vi "To String.vi"(8 "error in (no error)":errorcluster, 11 "BuildWorker in":refnum<class "BuildWorker.lvclass">) -> (0 "error out":errorcluster, 2 "String":string, 3 "BuildWorker out":refnum<class "BuildWorker.lvclass">)   [LabVIEW 2017, in "BuildWorker Interface.lvlib" / "BuildWorker.lvclass"]
uses:
  BuildWorker.lvclass
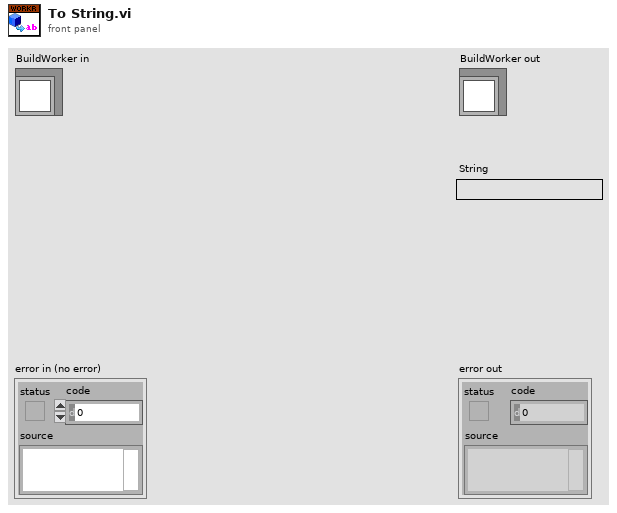
[diagram p1: front panel]
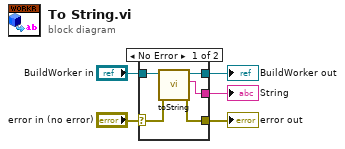
[diagram p0: block diagram]
diagram:
  n1 = case shown="No Error" "error in (no error)" {
    selector: "error in (no error)" -> [w8 w12]
    tunnel: [w7 w12] -> w4
    tunnel: [w9 w11] -> w2
    tunnel: "BuildWorker in" -> [w10 w11]
    tunnel: [w6 _] -> w1
    frame No Error {
      n2 = call-dynamic "toString.vi"("error in (no error)"=w8, "BuildWorker in"=w10) -> ("error out"=w7:errorcluster, "String"=w6:string, "BuildWorker out"=w9:refnum<class "BuildWorker.lvclass">)  [unwired: 7 in]
    }
    frame Error {
    }
  }
  "error out" <- w4
  "BuildWorker out" <- w2
  "String" <- w1
